vi "Bitfile Component Check.vi"(2 "error in (no error)":errorcluster, 3 "Control Scalars":T1) -> (0 "error out":errorcluster, 1 "Valid?":bool)   [LabVIEW 2012, in "AIT 429 System Explorer.lvlib"]
uses:
  AIT 429 System Explorer.lvlib
  <userlib>/_FPGA Interface Advanced Tools/FPGA Bitfile Utility/TypeDefs/Scalar Register Set.ctl
  <userlib>/_FPGA Interface Advanced Tools/FPGA Bitfile Utility/TypeDefs/Scalar Register.ctl
  <userlib>/_FPGA Interface Advanced Tools/FPGA Bitfile Utility/FPGA Bitfile Utility.lvlib
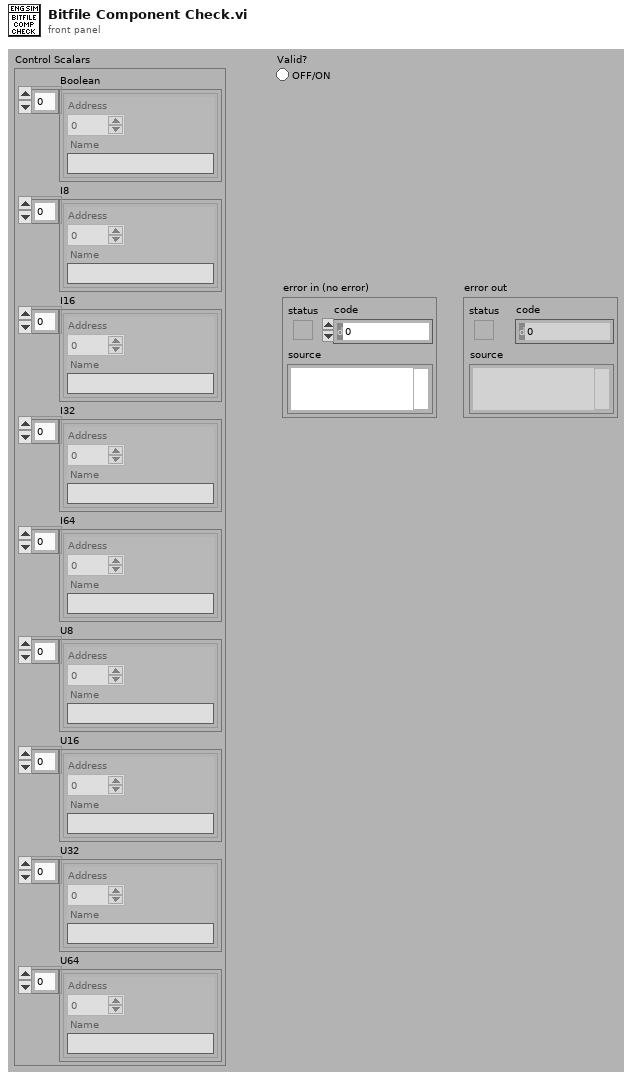
[diagram p1: front panel]
types:
  T1 = typedef "FPGA Bitfile Utility.lvlib/Scalar Register Set.ctl" = cluster{"Boolean":T2[], "I8":T2[], "I16":T2[], "I32":T2[], "I64":T2[], "U8":T2[], "U16":T2[], "U32":T2[], "U64":T2[]}
  T2 = typedef "FPGA Bitfile Utility.lvlib/Scalar Register.ctl" = cluster{"Address":u32, "Name":string}
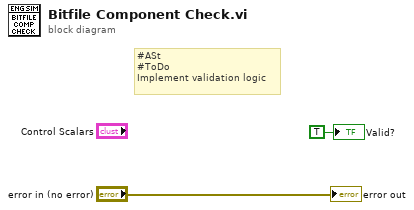
[diagram p0: block diagram]
diagram:
  # "#ASt\n#ToDo\nImplement validation logic"
  "Valid?" <- TRUE ("Valid?")
  "error out" <- "error in (no error)"
